vi "Write Call Back VI.vi"(8 "error in (no error)":errorcluster, 10 "Call Back VI":T1, 11 "Column in":refnum<class "Column.lvclass">) -> (0 "error out":errorcluster, 3 "Column out":refnum<class "Column.lvclass">)   [LabVIEW 2013, in "Table Manager.lvlib" / "Column.lvclass"]
uses:
  Column.lvclass
  Table Manager/Call Back Ref Type Def.ctl
  Configuration Editor/Classes/Engine Parent/Engine Parent Editor Node.lvclass
  Column.lvclass/Column.ctl
  Table Manager/Table Manager.lvclass
  Configuration Editor/Classes/Module editor node/module editor node.lvclass
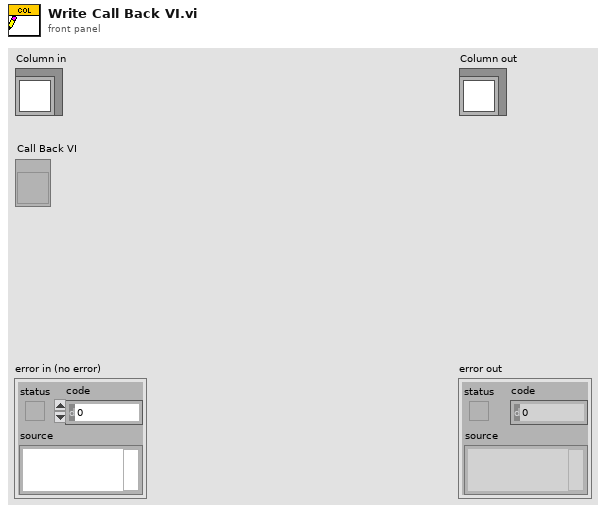
[diagram p1: front panel]
types:
  T1 = typedef "Table Manager.lvlib/Table Manager.lvclass/Call Back Ref Type Def.ctl" = refnum<vi>
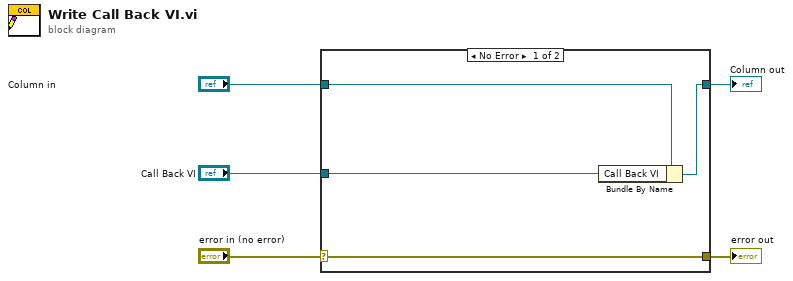
[diagram p0: block diagram]
diagram:
  n1 = case shown="No Error" "error in (no error)" {
    selector: "error in (no error)" -> [w9 w10]
    tunnel: [w9 w10] -> w4
    tunnel: [w7 w11] -> w2
    tunnel: "Column in" -> [w8 w11]
    tunnel: "Call Back VI" -> [w6 _]
    frame No Error {
      n2 = Bundle By Name(cluster=w8, "Call Back VI"=w6) -> (w7:refnum<class "Column.lvclass">)
    }
    frame Error {
    }
  }
  "error out" <- w4
  "Column out" <- w2
